vi "Teleop.vi"(10 "Match Info":T2={"Autonomous Elapsed Seconds"=0.0, "TeleOp Elapsed Seconds"=0.0, "Disabled Elapsed Seconds"=0.0, "Visited Autonomous"=FALSE, "Visited TeleOp"=FALSE, "Visited Disabled"=FALSE, "Autonomous Settings"={"Autonomous Style"=enum."Independent", "VI Refnum"=refnum}}, 11 "Call Context":T3) -> ()   [LabVIEW 2018]
doc: "This VI is called for each TeleOp packet received from the DS where the robot is not disabled. It is often used to read from the joysticks and update I/O or to update setpoints for timed control loops. It should complete and return within 20 milliseconds or it may miss DS packets."
uses:
  <vilib>/Rock Robotics/WPI/DriverStation/WPI_DriverStationDerivedRobotMode.ctl
  <vilib>/Rock Robotics/WPI/DriverStation/WPI_DriverStationMatch Info.ctl
  <vilib>/Rock Robotics/WPI/Solenoid/WPI_SolenoidValue.ctl
  <vilib>/Rock Robotics/WPI/Utilities/WPI_GetSetVariantRefNum.vi
  <vilib>/Rock Robotics/WPI/RobotDrive/WPI_RobotDriveMecanumDrive_Cartesian.vi
  <vilib>/Rock Robotics/WPI/RobotDrive/WPI_RobotDriveArcadeDrive_Standard(NoSaturation).vi
  <vilib>/Rock Robotics/WPI/Solenoid/WPI_SolenoidSetEnum.vi
panel:
  out "Modify Hoist":dbl
  out "Limit Switch":bool
  out "Suction Solenoid Value":T1
  out "Suction Button Pressed":dbl
  out "Tilt Solenoid Value":T1=enum."Forward"
  out "Tilt Button Pressed":dbl
  out "Y value 2":dbl
  out "Z value":dbl
  out "Y value":dbl
  out "X value":dbl
  out "Button 11\nSuction Push Out":bool
  out "Button 9\nSuction Off":bool
  out "Button 7\nSuction Pull In":bool
  out "Button 5\nTilt Up":bool
  out "Button 3\nTilt Down":bool
  # "Drive Control"
  # "Hoist Control"
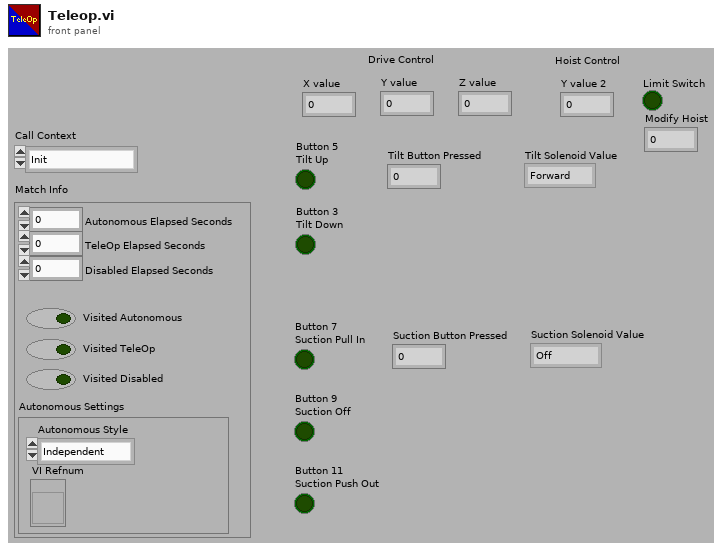
[diagram p1: front panel]
types:
  T1 = typedef "WPI_SolenoidValue.ctl" = enum16{"Off", "On", "Forward", "Reverse"}
  T2 = typedef "WPI_DriverStationMatch Info.ctl" = cluster{"Autonomous Elapsed Seconds":dbl, "TeleOp Elapsed Seconds":dbl, "Disabled Elapsed Seconds":dbl, "Visited Autonomous":bool, "Visited TeleOp":bool, "Visited Disabled":bool, "Autonomous Settings":cluster{"Autonomous Style":enum16{"Iterative", "Independent"}, "VI Refnum":refnum<vi>}}
  T3 = typedef "WPI_DriverStationDerivedRobotMode.ctl" = enum16{"Init", "Execute", "Stop"}
  T4 = typedef "WPI_DigitalInputDevRef.ctl" = cluster{"DevStatus":errorcluster, "DIO Channel":T5}
  T5 = typedef "FPGA_DIOChannel.ctl" = enum8{"DIO 0", "DIO 1", "DIO 2", "DIO 3", "DIO 4", "DIO 5", "DIO 6", "DIO 7", "DIO 8", "DIO 9", "DIO MXP 0", "DIO MXP 1", "DIO MXP 2", "DIO MXP 3", "DIO MXP 4", "DIO MXP 5", "DIO MXP 6", "DIO MXP 7", "DIO MXP 8", "DIO MXP 9", "DIO MXP 10", "DIO MXP 11", "DIO MXP 12", "DIO MXP 13", "DIO MXP 14", "DIO MXP 15", "SPI Port CS1", "SPI Port CS2", "SPI Port CS3", "SPI Port MISO", "SPI Port MOSI", "Invalid"}
  T6 = typedef "WPI_JoystickDevRef.ctl" = cluster{"Device":T7}
  T7 = typedef "WPI_JoystickDeviceEnum.ctl" = enum16{"USB 0", "USB 1", "USB 2", "USB 3", "USB 4", "USB 5"}
  T8 = typedef "WPI_RobotDriveDevRef.ctl" = cluster{"DevStatus":errorcluster, "Motors[]":T9[], "Square Inputs":bool, "Max Output":dbl}
  T9 = typedef "WPI_MotorControlDeviceRef.ctl" = cluster{"DeviceStatus":errorcluster, "Type":T10, "PWM":cluster{"PWM Channel":T11, "DeadBand":T12}, "CAN":cluster{"Device Number":u8, "SetOutput VI Ref":variant, "GetOutput VI Ref":variant, "Enable VI Ref":variant, "Disable VI Ref":variant, "Data":variant}, "Invert":bool, "DIO PWM":cluster{"PWM \"Enable\" Channel":T11, "DIOChannel":T5, "PWM Rate":dbl}}
  T10 = typedef "WPI_MotorControlType.ctl" = enum16{"PWM", "CAN", "DIO PWM"}
  T11 = typedef "FPGA_DIOPWMChannel.ctl" = enum8{"PWM 0", "PWM 1", "PWM 2", "PWM 3", "PWM 4", "PWM 5", "PWM 6", "PWM 7", "PWM 8", "PWM 9", "PWM MXP 0", "PWM MXP 1", "PWM MXP 2", "PWM MXP 3", "PWM MXP 4", "PWM MXP 5", "PWM MXP 6", "PWM MXP 7", "PWM MXP 8", "PWM MXP 9", "Invalid"}
  T12 = typedef "WPI_PWMDeadband.ctl" = cluster{"Name":string, "maxPositivePwm":i32, "minPositivePwm":i32, "centerPwm":i32, "maxNegativePwm":i32, "minNegativePwm":i32, "angularRange":u16}
  T13 = typedef "WPI_SolenoidDevRef.ctl" = cluster{"DevStatus":errorcluster, "Pneumatics Control Module":u8, "Forward Solenoid Channel":T14, "Reverse Solenoid Channel":T14}
  T14 = typedef "WPI_SolenoidChannel.ctl" = enum8{"Solenoid 0", "Solenoid 1", "Solenoid 2", "Solenoid 3", "Solenoid 4", "Solenoid 5", "Solenoid 6", "Solenoid 7", "Invalid"}
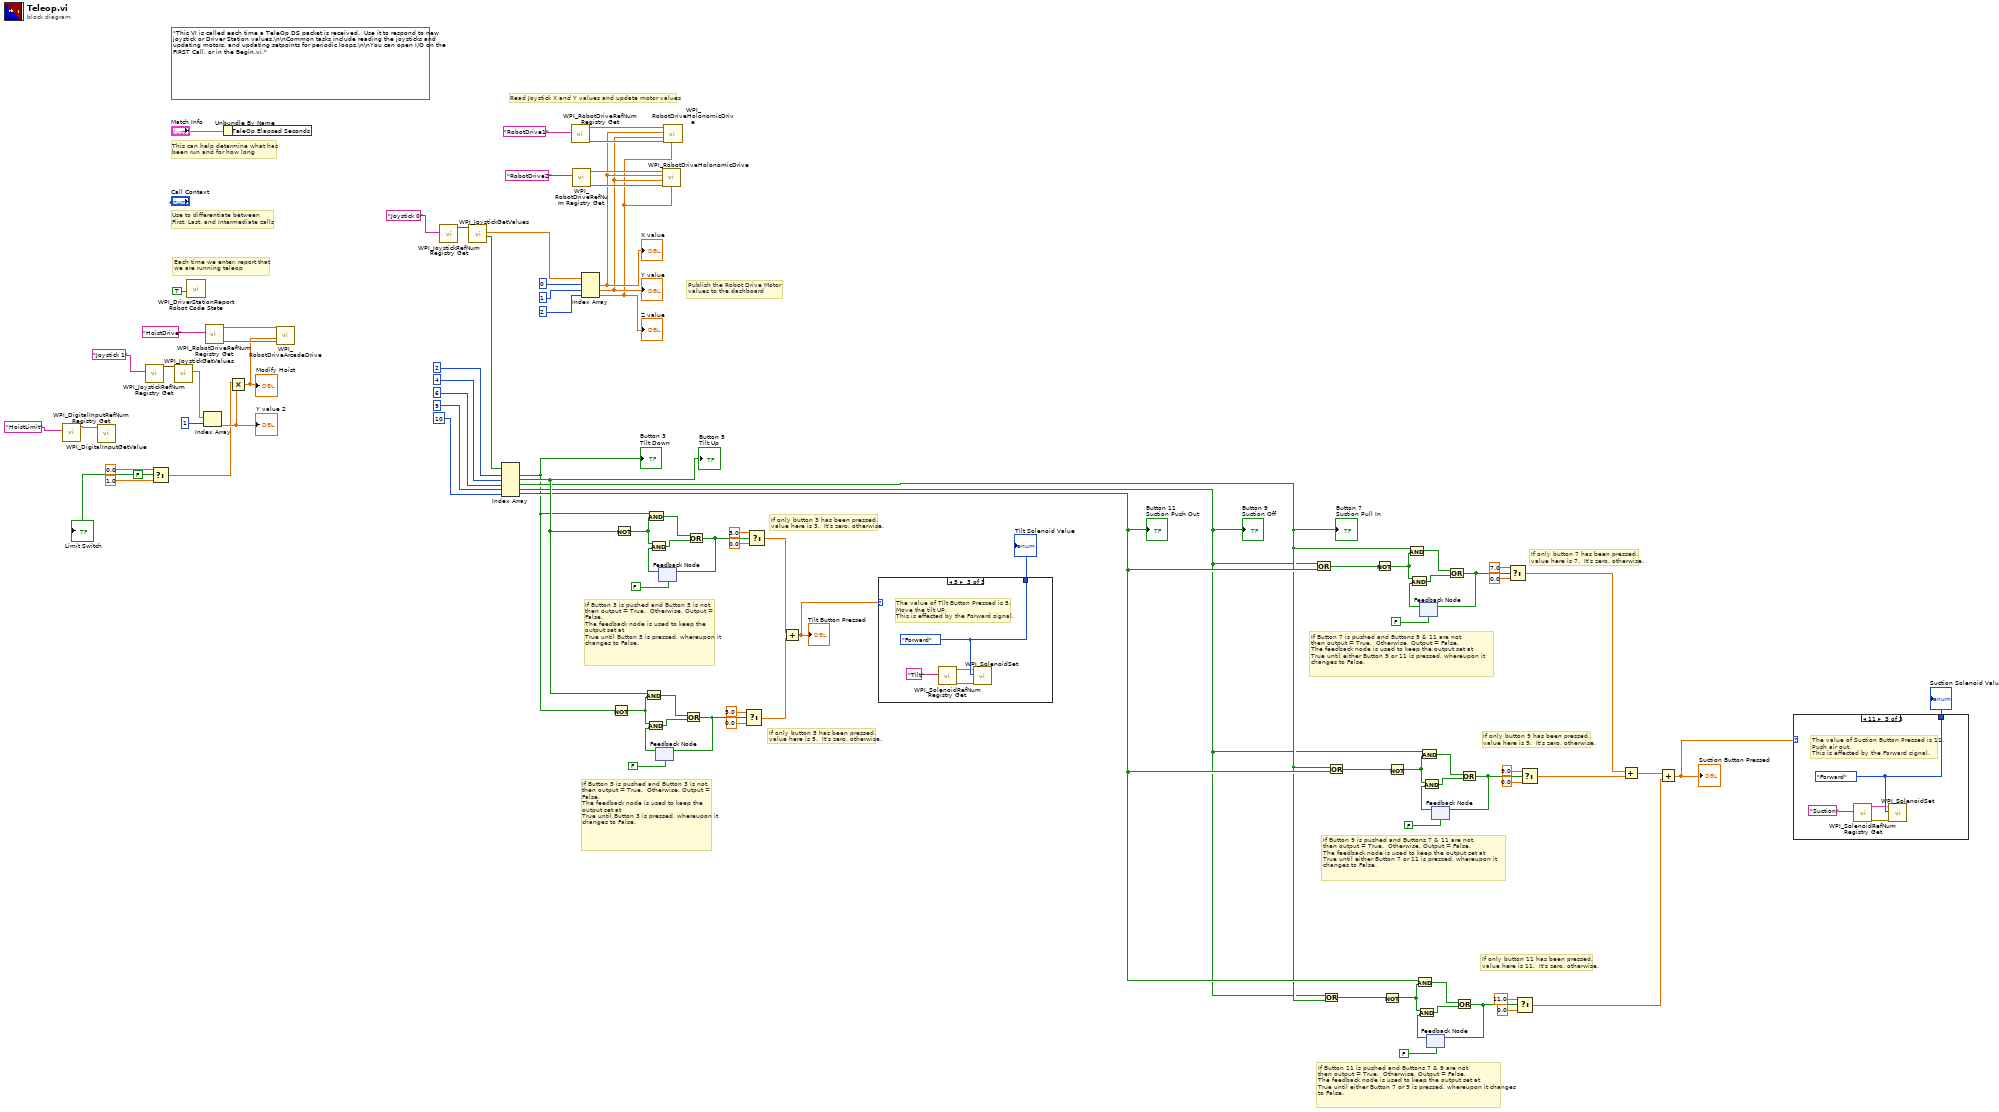
[diagram p0: block diagram]
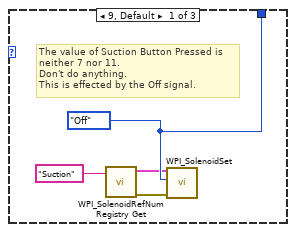
[diagram p2: hidden frame]
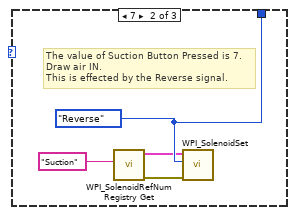
[diagram p3: hidden frame]
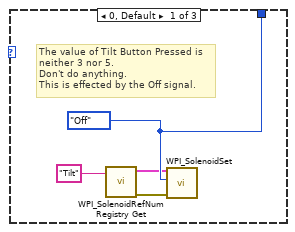
[diagram p4: hidden frame]
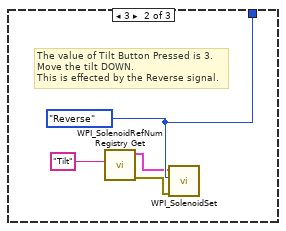
[diagram p5: hidden frame]
diagram:
  w1 = FALSE ("s")
  (unwired) "This VI is called each time a TeleOp DS packet is received.  Use it to respond to new joystick or Driver Station values.\n\nCommon tasks include reading the joysticks and updating motors, and updating setpoints for periodic loops.\n\nYou can open I/O on the FIRST Call, or in the Begin.vi."
  # "If only button 11 has been pressed,\nvalue here is 11.  It's zero, otherwise."
  # "If Button 11 is pushed and Buttons 7 & 9 are not,\nthen output = True.  Otherwise, Output = False.\nThe feedback node is used to keep the output set at \nTrue until either Button 7 or 9 is pressed, whereupon it changes to False."
  # "If only button 9 has been pressed,\nvalue here is 9.  It's zero, otherwise."
  # "If Button 9 is pushed and Buttons 7 & 11 are not,\nthen output = True.  Otherwise, Output = False.\nThe feedback node is used to keep the output set at \nTrue until either Button 7 or 11 is pressed, whereupon it changes to False."
  # "If only button 7 has been pressed,\nvalue here is 7.  It's zero, otherwise."
  # "If Button 7 is pushed and Buttons 9 & 11 are not,\nthen output = True.  Otherwise, Output = False.\nThe feedback node is used to keep the output set at \nTrue until either Button 9 or 11 is pressed, whereupon it changes to False."
  # "If only button 5 has been pressed,\nvalue here is 5.  It's zero, otherwise."
  # "If only button 3 has been pressed,\nvalue here is 3.  It's zero, otherwise."
  # "If Button 5 is pushed and Button 3 is not,\nthen output = True.  Otherwise, Output = False.\nThe feedback node is used to keep the output set at \nTrue until Button 3 is pressed, whereupon it changes to False."
  # "If Button 3 is pushed and Button 5 is not,\nthen output = True.  Otherwise, Output = False.\nThe feedback node is used to keep the output set at \nTrue until Button 5 is pressed, whereupon it changes to False."
  # "Publish the Robot Drive Motor\nvalues to the dashboard"
  # "Each time we enter, report that\nwe are running teleop"
  # "Use to differentiate between\nFirst, Last, and Intermediate calls"
  # "This can help determine what has\nbeen run and for how long"
  # "Read Joystick X and Y values and update motor values"
  n1 = call <vilib>:"WPI_DigitalInputRefNum Registry Get.vi"("refnum name"="HoistLimit") -> ("DigitalInputDevRef"=w2:T4)  [unwired: 9 in, 1 out]
  n2 = call <vilib>:"WPI_DigitalInputGetValue.vi"("DigitalInputDevRef"=w2) -> ()  [unwired: 8 in, 3 out]
  n3 = call <vilib>:"WPI_JoystickRefNum Registry Get.vi"("refnum name"="Joystick 1") -> ("JoystickDevRef"=w81:T6)  [unwired: 1 in, 9 out]
  n4 = Select(t=0.0, s=w1, f=1.0) -> (s? t:f=w6:dbl)
  n5 = call <vilib>:"WPI_JoystickGetValues.vi"("JoystickDevRef"=w81) -> ("Axes"=w80:dbl[])  [unwired: 6 in, 4 out]
  n6 = call <vilib>:"WPI_DriverStationReport Robot Code State.vi"("TeleOp"=TRUE ("Autonomous")) -> ()  [unwired: 10 in, 1 out]
  n7 = Index Array(array=w80, index=1) -> (element=w66:dbl)
  "Y value 2" <- w66
  n8 = call <vilib>:"WPI_RobotDriveRefNum Registry Get.vi"("refnum name"="HoistDrive") -> ("error out"=w67:errorcluster, "RobotDriveDevRef"=w68:T8)  [unwired: 9 in]
  n9 = Unbundle By Name("Match Info") -> ()  [unwired: 1 out]
  n10 = Multiply(x=w6, y=w66) -> (x*y=w7:dbl)
  "Modify Hoist" <- w7
  n11 = call-poly <vilib>:"WPI_RobotDriveArcadeDrive.vi"("error in (no error)"=w67, "Y axis value"=w7, "RobotDriveDevRef"=w68) -> ()  [unwired: 6 in, 3 out]
  n12 = call <vilib>:"WPI_JoystickRefNum Registry Get.vi"("refnum name"="Joystick 0") -> ("JoystickDevRef"=w94:T6)  [unwired: 1 in, 9 out]
  n13 = call <vilib>:"WPI_JoystickGetValues.vi"("JoystickDevRef"=w94) -> ("Buttons"=w91:bool[], "Axes"=w92:dbl[])  [unwired: 6 in, 3 out]
  n14 = Index Array(array=w91, index #1=2 ("index"), index #2=4 ("index"), index #3=6 ("index"), index #4=9 ("index"), index #5=10 ("index")) -> (element #1=w8:bool, element #2=w45:bool, element #3=w10:bool, element #4=w9:bool, element #5=w11:bool)
  "Button 3\nTilt Down" <- w8
  "Button 5\nTilt Up" <- w45
  "Button 7\nSuction Pull In" <- w10
  "Button 9\nSuction Off" <- w9
  "Button 11\nSuction Push Out" <- w11
  n15 = call <vilib>:"WPI_RobotDriveRefNum Registry Get.vi"("refnum name"="RobotDrive1") -> ("error out"=w76:errorcluster, "RobotDriveDevRef"=w77:T8)  [unwired: 9 in]
  n16 = call <vilib>:"WPI_RobotDriveRefNum Registry Get.vi"("refnum name"="RobotDrive2") -> ("error out"=w73:errorcluster, "RobotDriveDevRef"=w74:T8)  [unwired: 9 in]
  n17 = Index Array(array=w92, index #1=0 ("index"), index #2=1 ("index"), index #3=2 ("index")) -> (element #1=w72:dbl, element #2=w71:dbl, element #3=w70:dbl)
  "X value" <- w72
  "Y value" <- w71
  "Z value" <- w70
  n18 = Not(x=w8) -> (.not. x?=w59:bool)
  n19 = Not(x=w45) -> (.not. x?=w65:bool)
  n20 = And(x=w45, y=w59) -> (x .and. y?=w58:bool)
  n21 = And(x=w8, y=w65) -> (x .and. y?=w64:bool)
  n22 = feedback #1(FALSE) -> (w56:bool)
  n23 = And(x=w59, y=w56) -> (x .and. y?=w57:bool)
  n24 = feedback #2(FALSE) -> (w62:bool)
  n25 = And(x=w65, y=w62) -> (x .and. y?=w63:bool)
  n26 = call-poly <vilib>:"WPI_RobotDriveHolonomicDrive.vi"("Rotation"=w70, "error in (no error)"=w73, "Y"=w71, "X"=w72, "RobotDriveDevRef"=w74) -> ()  [unwired: 4 in, 3 out]
  n27 = call-poly <vilib>:"WPI_RobotDriveHolonomicDrive.vi"("Rotation"=w70, "error in (no error)"=w76, "Y"=w71, "X"=w72, "RobotDriveDevRef"=w77) -> ()  [unwired: 4 in, 3 out]
  n28 = Or(x=w58, y=w57) -> (x .or. y?=w54:bool)
  n29 = feedback-in #1(w54) -> ()
  n30 = Or(x=w64, y=w63) -> (x .or. y?=w60:bool)
  n31 = feedback-in #2(w60) -> ()
  n32 = Select(t=5.0, s=w54, f=0.0) -> (s? t:f=w48:dbl)
  n33 = Select(t=3.0, s=w60, f=0.0) -> (s? t:f=w49:dbl)
  n34 = Add(x=w49, y=w48) -> (x+y=w47:dbl)
  "Tilt Button Pressed" <- w47
  n35 = case shown="5" w47 {
    tunnel: [w100 w104 w108] -> w46
    frame 0, Default {
      w100 = WPI_SolenoidValue."Off" ("Value")
      # "The value of Tilt Button Pressed is \nneither 3 nor 5.\nDon't do anything.\nThis is effected by the Off signal."
      n36 = call <vilib>:"WPI_SolenoidRefNum Registry Get.vi"("refnum name"="Tilt") -> ("error out"=w99:errorcluster, "SolenoidDevRef"=w98:T13)  [unwired: 9 in]
      n37 = call-poly <vilib>:"WPI_SolenoidSet.vi"("error in (no error)"=w99, "Value"=w100, "SolenoidDevRef"=w98) -> ()  [unwired: 7 in, 2 out]
    }
    frame 3 {
      w104 = WPI_SolenoidValue."Reverse" ("Value")
      # "The value of Tilt Button Pressed is 3.\nMove the tilt DOWN.\nThis is effected by the Reverse signal."
      n38 = call <vilib>:"WPI_SolenoidRefNum Registry Get.vi"("refnum name"="Tilt") -> ("error out"=w101:errorcluster, "SolenoidDevRef"=w102:T13)  [unwired: 9 in]
      n39 = call-poly <vilib>:"WPI_SolenoidSet.vi"("error in (no error)"=w101, "Value"=w104, "SolenoidDevRef"=w102) -> ()  [unwired: 7 in, 2 out]
    }
    frame 5 {
      w108 = WPI_SolenoidValue."Forward" ("Value")
      # "The value of Tilt Button Pressed is 5.\nMove the tilt UP.\nThis is effected by the Forward signal."
      n40 = call <vilib>:"WPI_SolenoidRefNum Registry Get.vi"("refnum name"="Tilt") -> ("error out"=w105:errorcluster, "SolenoidDevRef"=w106:T13)  [unwired: 9 in]
      n41 = call-poly <vilib>:"WPI_SolenoidSet.vi"("error in (no error)"=w105, "Value"=w108, "SolenoidDevRef"=w106) -> ()  [unwired: 7 in, 2 out]
    }
  }
  "Tilt Solenoid Value" <- w46
  n42 = Or(x=w9, y=w11) -> (x .or. y?=w35:bool)
  n43 = Or(x=w9, y=w10) -> (x .or. y?=w17:bool)
  n44 = Or(x=w10, y=w11) -> (x .or. y?=w26:bool)
  n45 = Not(x=w35) -> (.not. x?=w44:bool)
  n46 = Not(x=w17) -> (.not. x?=w25:bool)
  n47 = Not(x=w26) -> (.not. x?=w34:bool)
  n48 = And(x=w10, y=w44) -> (x .and. y?=w43:bool)
  n49 = And(x=w11, y=w25) -> (x .and. y?=w24:bool)
  n50 = feedback #3(FALSE) -> (w41:bool)
  n51 = And(x=w44, y=w41) -> (x .and. y?=w42:bool)
  n52 = And(x=w9, y=w34) -> (x .and. y?=w33:bool)
  n53 = feedback #4(FALSE) -> (w22:bool)
  n54 = And(x=w25, y=w22) -> (x .and. y?=w23:bool)
  n55 = feedback #5(FALSE) -> (w31:bool)
  n56 = And(x=w34, y=w31) -> (x .and. y?=w32:bool)
  n57 = Or(x=w43, y=w42) -> (x .or. y?=w39:bool)
  n58 = feedback-in #3(w39) -> ()
  n59 = Or(x=w24, y=w23) -> (x .or. y?=w20:bool)
  n60 = feedback-in #4(w20) -> ()
  n61 = Or(x=w33, y=w32) -> (x .or. y?=w29:bool)
  n62 = feedback-in #5(w29) -> ()
  n63 = Select(t=7.0, s=w39, f=0.0) -> (s? t:f=w36:dbl)
  n64 = Select(t=11.0, s=w20, f=0.0) -> (s? t:f=w14:dbl)
  n65 = Select(t=9.0, s=w29, f=0.0) -> (s? t:f=w16:dbl)
  n66 = Add(x=w36, y=w16) -> (x+y=w15:dbl)
  n67 = Add(x=w15, y=w14) -> (x+y=w13:dbl)
  "Suction Button Pressed" <- w13
  n68 = case shown="11" w13 {
    tunnel: [w112 w116 w120] -> w12
    frame 9, Default {
      w112 = WPI_SolenoidValue."Off" ("Value")
      # "The value of Suction Button Pressed is \nneither 7 nor 11.\nDon't do anything.\nThis is effected by the Off signal."
      n69 = call <vilib>:"WPI_SolenoidRefNum Registry Get.vi"("refnum name"="Suction") -> ("error out"=w111:errorcluster, "SolenoidDevRef"=w110:T13)  [unwired: 9 in]
      n70 = call-poly <vilib>:"WPI_SolenoidSet.vi"("error in (no error)"=w111, "Value"=w112, "SolenoidDevRef"=w110) -> ()  [unwired: 7 in, 2 out]
    }
    frame 7 {
      w116 = WPI_SolenoidValue."Reverse" ("Value")
      # "The value of Suction Button Pressed is 7.\nDraw air IN.\nThis is effected by the Reverse signal."
      n71 = call <vilib>:"WPI_SolenoidRefNum Registry Get.vi"("refnum name"="Suction") -> ("error out"=w113:errorcluster, "SolenoidDevRef"=w114:T13)  [unwired: 9 in]
      n72 = call-poly <vilib>:"WPI_SolenoidSet.vi"("error in (no error)"=w113, "Value"=w116, "SolenoidDevRef"=w114) -> ()  [unwired: 7 in, 2 out]
    }
    frame 11 {
      w120 = WPI_SolenoidValue."Forward" ("Value")
      # "The value of Suction Button Pressed is 11.\nPush air out.\nThis is effected by the Forward signal."
      n73 = call <vilib>:"WPI_SolenoidRefNum Registry Get.vi"("refnum name"="Suction") -> ("error out"=w117:errorcluster, "SolenoidDevRef"=w118:T13)  [unwired: 9 in]
      n74 = call-poly <vilib>:"WPI_SolenoidSet.vi"("error in (no error)"=w117, "Value"=w120, "SolenoidDevRef"=w118) -> ()  [unwired: 7 in, 2 out]
    }
  }
  "Suction Solenoid Value" <- w12
  "Limit Switch" <- w1
